vi "detach_listener.vi"(8 "error in (no error)":errorcluster, 10 "listener":refnum<class "GenericToplevelComponent.lvclass">, 11 "GenericImageAssembler in":refnum<class "GenericImageAssembler.lvclass">) -> (0 "error out":errorcluster, 3 "GenericImageAssembler out":refnum<class "GenericImageAssembler.lvclass">)   [LabVIEW 2010]
uses:
  common/classes/Image/Image/Image.lvclass
  common/classes/GenericToplevelComponent/GenericToplevelComponent/GenericToplevelComponent.lvclass
  common/classes/GenericComponent/GenericComponent/GenericComponent.lvclass
  GenericImageAssembler.lvclass
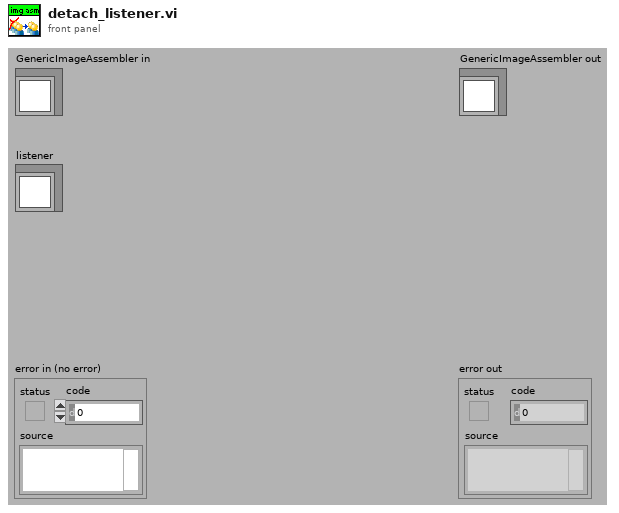
[diagram p1: front panel]
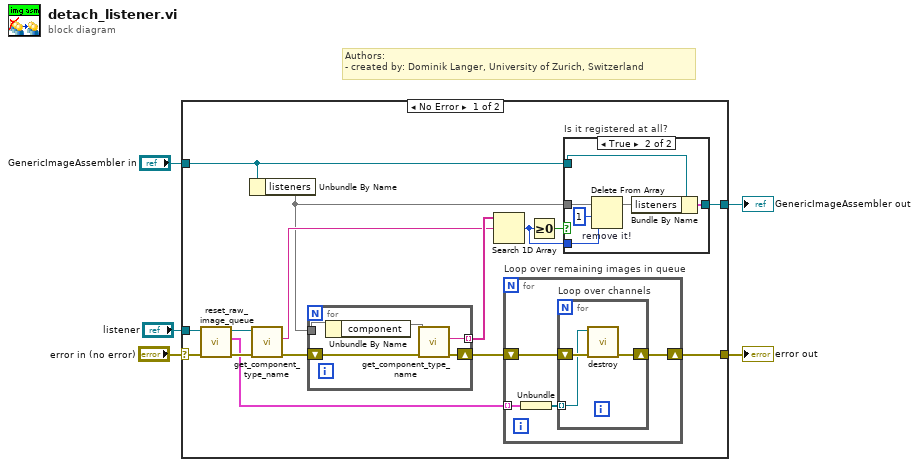
[diagram p0: block diagram]
diagram:
  # "Authors: \n- created by: Dominik Langer, University of Zurich, Switzerland"
  n1 = case shown="No Error" "error in (no error)" {
    selector: "error in (no error)" -> [w11 w41]
    tunnel: [w13 w41] -> w4
    tunnel: [w16 w40] -> w2
    tunnel: "GenericImageAssembler in" -> [w17 w40]
    tunnel: "listener" -> [w10 _]
    frame No Error {
      n2 = call-dynamic "reset_raw_image_queue.vi"("error in (no error)"=w11, "GenericToplevelComponent in"=w10) -> ("error out"=w9:errorcluster, "remaining elements"=w6:cluster{refnum<class "Image.lvclass">[]}[], "GenericToplevelComponent out"=w8:refnum<class "GenericToplevelComponent.lvclass">)  [unwired: 7 in]
      n3 = Unbundle By Name(w17) -> ("listeners"=w18)
      n4 = call-dynamic "get_component_type_name.vi"("error in (no error)"=w9, "GenericPlugin in"=w8) -> ("error out"=w12:errorcluster, "component type"=w19:string)  [unwired: 7 in, 1 out]
      n5 = for {
        shift-right: [w38] -> w7
        shift-left: w12 -> [w39]
        tunnel: w18 -> [w36]
        tunnel: [w37] -> w20 mode=indexing
        n6 = Unbundle By Name(w36) -> ("component"=w35)
        n7 = call-dynamic "get_component_type_name.vi"("error in (no error)"=w39, "GenericPlugin in"=w35) -> ("error out"=w38:errorcluster, "component type"=w37:string)  [unwired: 7 in, 1 out]
      }
      n8 = Search 1D Array(1D array=w20, element=w19) -> (index of element=w14:i32)  [unwired: 1 in]
      n9 = for "Loop over remaining images in queue" {
        tunnel: w6 -> [w24] mode=indexing
        shift-right: [w21] -> w13
        shift-left: w7 -> [w23]
        n10 = Unbundle(w24) -> (w22:refnum<class "Image.lvclass">[])
        n11 = for "Loop over channels" {
          tunnel: w22 -> [w26] mode=indexing
          shift-right: [w25] -> w21
          shift-left: w23 -> [w27]
          n12 = call-dynamic "destroy.vi"("error in (no error)"=w27, "Image in"=w26) -> ("error out"=w25:errorcluster)  [unwired: 9 out]
        }
      }
      n13 = Greater Or Equal To 0?(x=w14) -> (x >= 0?=w15:bool)
      n14 = case "Is it registered at all?" shown="True" w15 {
        tunnel: w18 -> [_ w34]
        tunnel: w17 -> [w28 w32]
        tunnel: [w28 w31] -> w16
        tunnel: w14 -> [_ w30]
        frame False {
          # "No action required..."
        }
        frame True {
          n15 = Delete From Array "remove it!"(array=w34, length=1, index=w30) -> (array with subset deleted=w33)  [unwired: 1 out]
          n16 = Bundle By Name(cluster=w32, "listeners"=w33) -> (w31:cluster{})
        }
      }
    }
    frame Error {
    }
  }
  "error out" <- w4
  "GenericImageAssembler out" <- w2
